vi "Create Base Tree.vi"(8 "error in (no error)":errorcluster, 10 "Root UID":string) -> (0 "error out":errorcluster, 3 "Base Tree out":refnum<class "Base Tree.lvclass">)   [LabVIEW 2017, in "Browser Core.lvlib" / "Base Tree.lvclass"]
doc: "Create Tree with Root UID defining the root node."
uses:
  Base Tree.lvclass
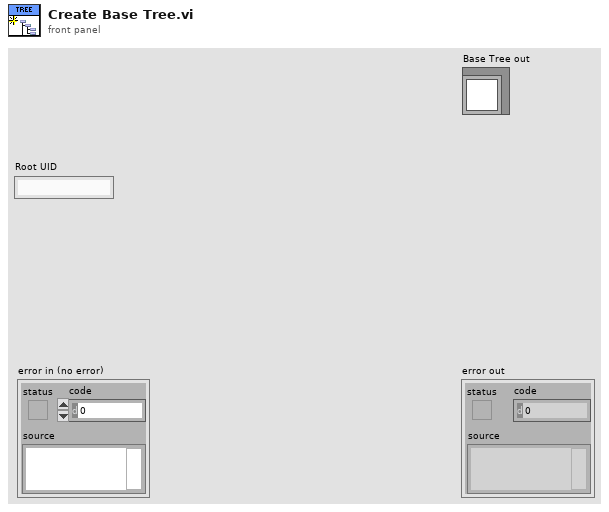
[diagram p1: front panel]
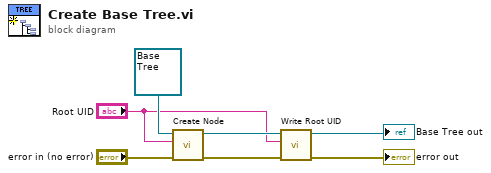
[diagram p0: block diagram]
diagram:
  n1 = call "Create Node.vi"("error in (no error)"="error in (no error)", "UID"="Root UID", "Base Tree in"=refnum<class "Base Tree.lvclass"> refnum ("Base Tree out")) -> ("error out"=w4:errorcluster, "Base Tree out"=w5:refnum<class "Base Tree.lvclass">)  [unwired: 7 in]
  n2 = call "Write Root UID.vi"("error in (no error)"=w4, "Root UID"="Root UID", "Base Tree in"=w5) -> ("error out"=→"error out":errorcluster, "Base Tree out"=→"Base Tree out":refnum<class "Base Tree.lvclass">)  [unwired: 7 in]
